vi "Read Time Waveforms with Records (UFF File).vi"() -> ()   [LabVIEW 2017]
doc: "Overview:\nThis VI demonstrates reading all time waveforms from a UFF58 data file.\n\nRequirements:\nLabVIEW Full Development System\nSound and Vibration Toolkit\n\nInstructions:\nRun the VI.\n\nDetails:\nThis example reads time waveforms and the associated records from a data file stored in the Universal File Format 58b (UFF 58b). This format is commonly used in structural analysis applications and stores header information in ASCII format and data in binary format."
uses:
  <vilib>/addons/Sound and Vibration/svt_UFF58/subVIs/sv_FunctionType.ctl
  <vilib>/addons/Sound and Vibration/svt_UFF58/subVIs/sv_UFF58 Specific Datatype.ctl
  <vilib>/addons/Sound and Vibration/svt_UFF58/subVIs/sv_UFF58 Response Direction.ctl
  <vilib>/addons/Sound and Vibration/svt_UFF58/subVIs/sv_UFF58 Open Mode.ctl
  <vilib>/addons/Sound and Vibration/svt_UFF58/subVIs/sv_UFF58 Get FunctionType.ctl
  <vilib>/addons/Sound and Vibration/svt_UFF58/SVT UFF58 Read Time Waveform.vi
  <vilib>/addons/Sound and Vibration/svt_UFF58/SoundVib_UFF58.lvlib
panel:
  out "Function \nnumber":T3(array[cluster]) {"response direction" items=["-Z Rotation"=-6, "-Y Rotation"=-5, "-X Rotation"=-4, "-Z Translation"=-3, "-Y Translation"=-2, "-X Translation"=-1, "Scalar"=0, "+X Translation"=1, "+Y Translation"=2, "+Z Translation"=3, "+X Rotation"=4, "+Y Rotation"=5, "+Z Rotation"=6]}
  out "number of time waveforms in the UFF file":i32
  out "Function details":T5(array[cluster]) {"specific data type 2" items=["unknown"=0, "general"=1, "stress"=2, "strain"=3, "temperature"=5, "heat flux"=6, "displacement"=8, "reaction force"=9, "velocity"=11, "acceleration"=12, "excitation force"=13, "pressure"=15, "mass"=16, "time"=17, "frequency"=18, "rpm"=19, "order"=20, "sound pressure"=21, "sound intensity"=22, "sound power"=23]; "specific data type" items=["unknown", "general", "stress", "strain", "temperature", "heat flux", "displacement", "reaction force", "velocity", "acceleration", "excitation force", "pressure", "mass", "time", "frequency", "rpm", "order"]}
  out "Time Waveforms":waveform(dbl)[](graph)
  in  "UFF58 file path to read":path
  # "UFF58 Details"
  # "UFF58 Data"
  # "Function \nnumber"
  # "Function \ntype"
  # "Number of\ndata pairs"
  # "Abscissa \ndatatype"
  # "Ordinate \ndatatype"
  # "Description"
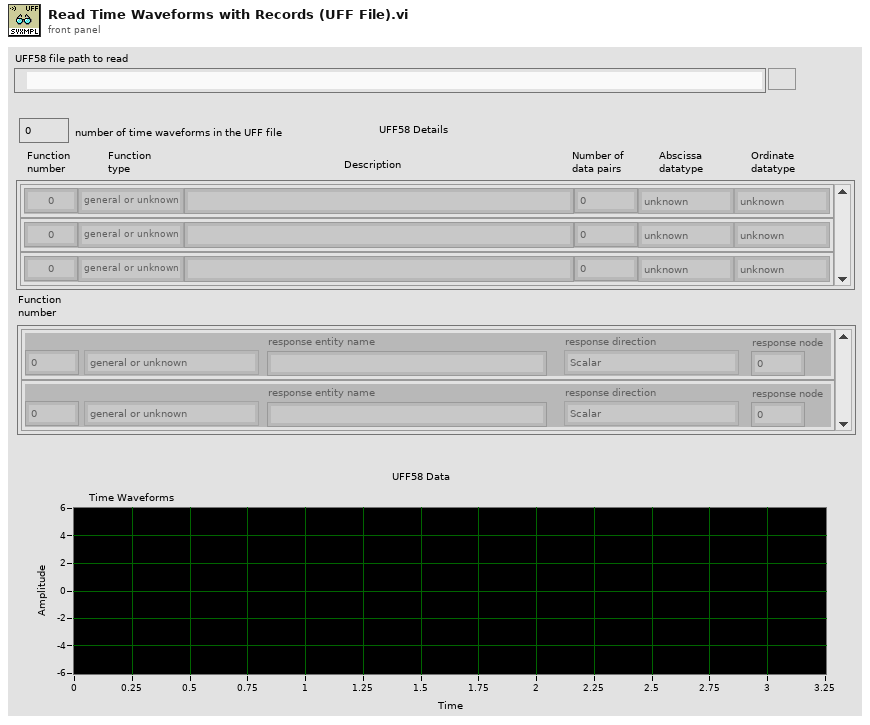
[diagram p1: front panel]
types:
  T1 = typedef "SoundVib_UFF58.lvlib/sv_FunctionType.ctl" = enum16{"general or unknown", "time response", "auto spectrum", "cross spectrum", "frequency response function", "transmissibility", "coherence", "auto correlation", "cross correlation", "power spectral density (PSD)", "energy spectral density (ESD)", "probability density function", "spectrum", "cumulative frequency distribution", "peaks valley", "stress/cycles", "strain/cycles", "orbit", "mode indicator function", "force pattern", "partial power", "partial coherence", "eigenvalue", "eigenvector", "shock response spectrum", "finite impulse response filter", "multiple coherence", "order function", "phase compensation"}
  T2 = typedef "SoundVib_UFF58.lvlib/sv_UFF58 Response Direction.ctl" = i32
  T3 = cluster{i32, "function type":T1, "response entity name":string, "response node":i32, "response direction":T2}[]
  T4 = typedef "SoundVib_UFF58.lvlib/sv_UFF58 Specific Datatype.ctl" = u16
  T5 = cluster{i32, "function type":T1, "ID line 1 (description)":string, "number of data values/pairs":i32, "specific data type 2":T4, "specific data type":T4}[]
  T6 = typedef "SoundVib_UFF58.lvlib/sv_UFF58 Get FunctionType.ctl" = enum16{"all functions", "all time waveforms", "all spectra (real)", "all spectra (complex)", "general or unknown", "time response", "auto spectrum", "cross spectrum", "frequency response function", "transmissibility", "coherence", "auto correlation", "cross correlation", "power spectral density (PSD)", "energy spectral density (ESD)", "probability density function", "spectrum", "cumulative frequency distribution", "peaks valley", "stress/cycles", "strain/cycles", "orbit", "mode indicator function", "force pattern", "partial power", "partial coherence", "eigenvalue", "eigenvector", "shock response spectrum", "finite impulse response filter", "multiple coherence", "order function"}
  T7 = typedef "SoundVib_UFF58.lvlib/sv_UFF58 Open Mode.ctl" = enum16{"create ", "create or replace", "open (read only)"}
  T8 = typedef "SoundVib_UFF58.lvlib/sv_IDLines123.ctl" = cluster{"ID line 1 (description)":string, "ID line 2":string, "ID line 3 (date & time)":string}
  T9 = typedef "SoundVib_UFF58.lvlib/sv_UFF58 DOF.ctl" = cluster{"function type":T1, "function ID number":i32, "version number":i32, "load case ID number":i32, "response entity name":string, "response node":i32, "response direction":T2, "reference entity name":string, "reference node":i32, "reference direction":T2}
  T10 = typedef "SoundVib_UFF58.lvlib/sv_UFF58 Data Form.ctl" = cluster{"ordinate data type":u16, "number of data values/pairs":i32, "abscissa spacing":enum16{"uneven", "even"}, "abscissa minimum":dbl, "abscissa increment":dbl}
  T11 = typedef "SoundVib_UFF58.lvlib/sv_UFF58 Axis Characteristics.ctl" = cluster{"specific data type":T4, "length units exponent":i32, "force units exponent":i32, "temperature units exponent":i32, "axis label":string, "axis units label":string}
  T12 = cluster{i32, "function type":T1, "ID line 1 (description)":string, "number of data values/pairs":i32, "specific data type":T4, "specific data type":T4}
  T13 = cluster{i32, "function type":T1, "response entity name":string, "response node":i32, "response direction":T2}
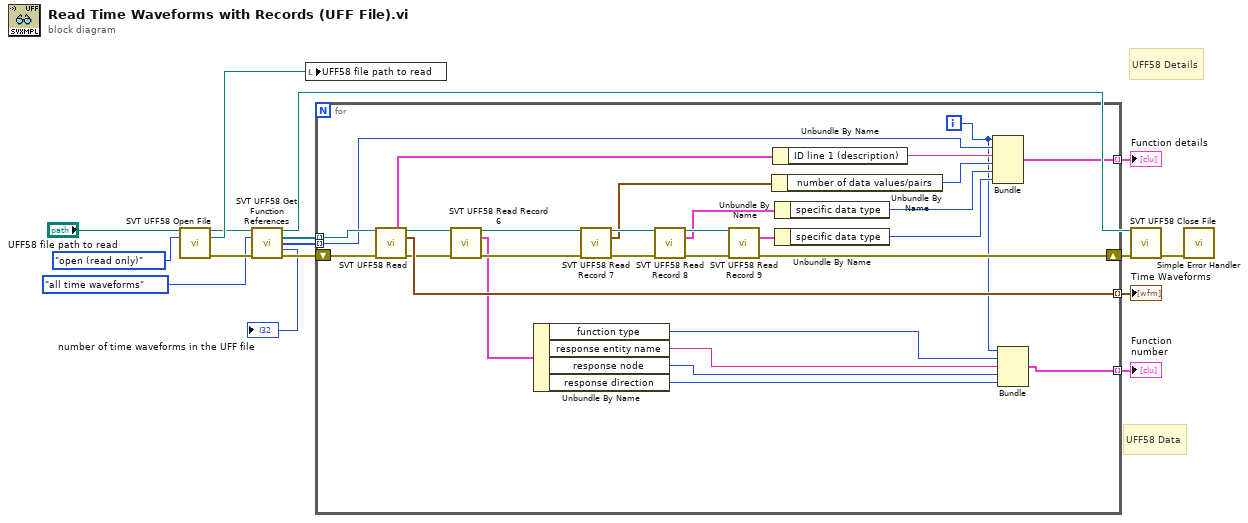
[diagram p0: block diagram]
diagram:
  # "UFF58 Details"
  # "UFF58 Data"
  n1 = call <vilib>:"SVT UFF58 Open File.vi"("UFF58 file path"="UFF58 file path to read", "open mode (create:0)"=sv_UFF58_Open_Mode."open (read only)") -> ("file refnum"=w4:refnum<k20>, "UFF58 file path out"=w16:path, "error out"=w14:errorcluster)  [unwired: 11 in]
  n2 = call <vilib>:"SVT UFF58 Get Function References.vi"("file refnum"=w4, "function type (all functions:0)"=sv_UFF58_Get_FunctionType."all time waveforms" ("Get function type"), "error in (no error)"=w14) -> ("dup file refnum"=w11:refnum<k20>, "function refnums"=w12:refnum<k20>[], "function types"=w2:T1[], "number of functions"=→"number of time waveforms in the UFF file":i32, "error out"=w13:errorcluster)  [unwired: 8 in]
  n3 = local write "UFF58 file path to read"(w16) -> ()
  n4 = for {
    shift-right: [w38] -> w15
    shift-left: w13 -> [w29]
    tunnel: w12 -> [w30] mode=indexing
    tunnel: [w44] -> w7 mode=indexing
    tunnel: [w33] -> w5 mode=indexing
    tunnel: w2 -> [w28] mode=indexing
    tunnel: [w18] -> w1 mode=indexing
    i -> [w19]
    n5 = call-poly <vilib>:"SVT UFF58 Read.vi"("function refnum"=w30, "error in (no error)"=w29) -> ("ID lines (1-3)"=w45:T8, "dup function refnum"=w27:refnum<k20>, "waveform"=w44:waveform(dbl), "error out"=w26:errorcluster)  [unwired: 10 in]
    n6 = call <vilib>:"SVT UFF58 Read Record 6.vi"("function refnum"=w27, "error in (no error)"=w26) -> ("dup function refnum"=w24:refnum<k20>, "DOF identification"=w17:T9, "error out"=w25:errorcluster)  [unwired: 11 in]
    n7 = Unbundle By Name(w17) -> ("function type"=w20:T1, "response entity name"=w21:string, "response node"=w22:i32, "response direction"=w23:T2)
    n8 = call <vilib>:"SVT UFF58 Read Record 7.vi"("function refnum"=w24, "error in (no error)"=w25) -> ("dup function refnum"=w39:refnum<k20>, "data form"=w31:T10, "error out"=w40:errorcluster)  [unwired: 11 in]
    n9 = call <vilib>:"SVT UFF58 Read Record 8.vi"("function refnum"=w39, "error in (no error)"=w40) -> ("dup function refnum"=w42:refnum<k20>, "abscissa data characteristics"=w37:T11, "error out"=w41:errorcluster)  [unwired: 11 in]
    n10 = call <vilib>:"SVT UFF58 Read Record 9.vi"("function refnum"=w42, "error in (no error)"=w41) -> ("ordinate data characteristics"=w36:T11, "error out"=w38:errorcluster)  [unwired: 11 in, 1 out]
    n11 = Unbundle By Name(w31) -> ("number of data values/pairs"=w43:i32)
    n12 = Unbundle By Name(w45) -> ("ID line 1 (description)"=w32:string)
    n13 = Unbundle By Name(w37) -> ("specific data type"=w35:T4)
    n14 = Unbundle By Name(w36) -> ("specific data type"=w34:T4)
    n15 = Bundle(w19, "function type"=w28, "ID line 1 (description)"=w32, "number of data values/pairs"=w43, "specific data type"=w35, "specific data type"=w34) -> (w33:T12)  [unwired: 1 in]
    n16 = Bundle(w19, "function type"=w20, "response entity name"=w21, "response node"=w22, "response direction"=w23) -> (w18:T13)  [unwired: 1 in]
  }
  "Time Waveforms" <- w7
  "Function details" <- w5
  "Function \nnumber" <- w1
  n17 = call <vilib>:"SVT UFF58 Close File.vi"("file refnum"=w11, "error in (no error)"=w15) -> ("error out"=w9:errorcluster)  [unwired: 13 in]
  n18 = call <vilib>:"Simple Error Handler.vi"("error in (no error)"=w9) -> ()  [unwired: 4 in, 5 out]
